vi "loadData.vi"(8 "error in (no error)":errorcluster, 10 "Data":T1={"Timestamps ms"=[0.0, 0.005, 0.009, 0.012], "DataPerChannel"=[]} {"Timestamps ms" format="%.3f"}, 11 "DigitalOutput in":refnum<class "DigitalOutput.lvclass">) -> (0 "error out":errorcluster, 3 "DigitalOutput out":refnum<class "DigitalOutput.lvclass">)   [LabVIEW 2009, in "Hardware.lvlib" / "Channels.lvlib" / "DigitalOutput.lvclass"]
uses:
  DigitalOutput.lvclass
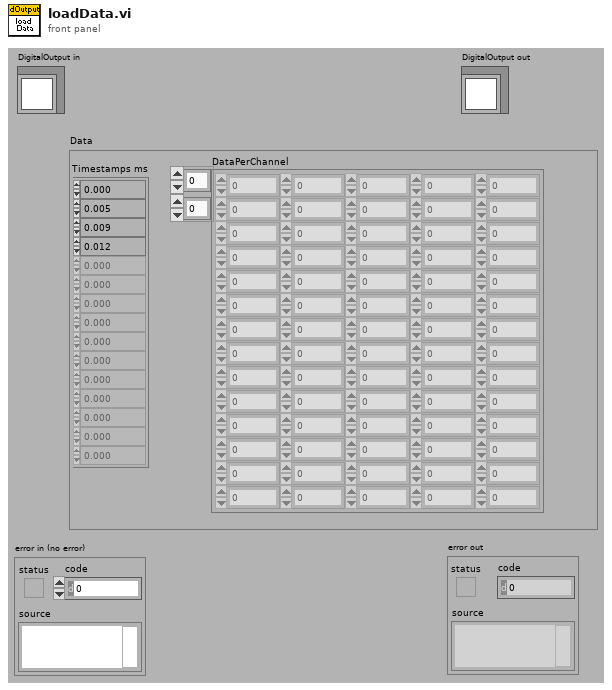
[diagram p1: front panel]
types:
  T1 = cluster{"Timestamps ms":dbl[], "DataPerChannel":dbl[][]}
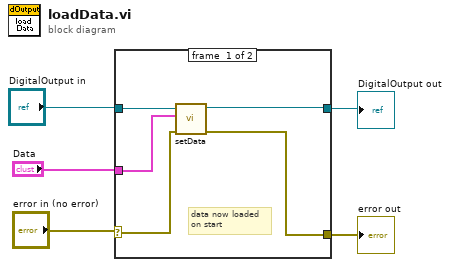
[diagram p0: block diagram]
diagram:
  n1 = case shown="No Error" "error in (no error)" {
    selector: "error in (no error)" -> [w8 w12]
    tunnel: [w6 w12] -> w4
    tunnel: [w7 w11] -> w2
    tunnel: "DigitalOutput in" -> [w10 w11]
    tunnel: "Data" -> [w9 _]
    frame #0 {
      # "data now loaded\non start"
      n2 = call-dynamic "setData.vi"("error in (no error)"=w8, "Data"=w9, "DigitalOutput.lvclass in"=w10) -> ("error out"=w6:errorcluster, "DigitalOutput.lvclass out"=w7:refnum<class "DigitalOutput.lvclass">)  [unwired: 7 in]
    }
    frame #1 {
    }
  }
  "error out" <- w4
  "DigitalOutput out" <- w2
